vi "Heartbeat Service.vi"() -> ()   [LabVIEW 2015]
doc: "This VeriStand service checks to see if the daemon associated with the Host Hearbeat custom device is running. If the daemon is running, the service does nothing. If the deamon isn't running, the service launches the daemon. The service checks daemon status only once then ends execution."
uses:
  NationalInstruments.VeriStand.SystemStorage
  Shared/Constants.vi
  Shared/Host Heartbeat Shared.lvlib
panel:
  in  "NIVS.System Definition Root":refnum<k24>
  in  "NIVS.Gateway IP Address":string
  # "These controls are written to by name when VeriStand \nlaunches the service. DO NOT modify their names"
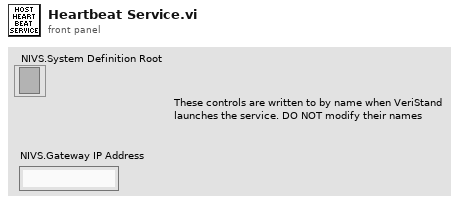
[diagram p1: front panel]
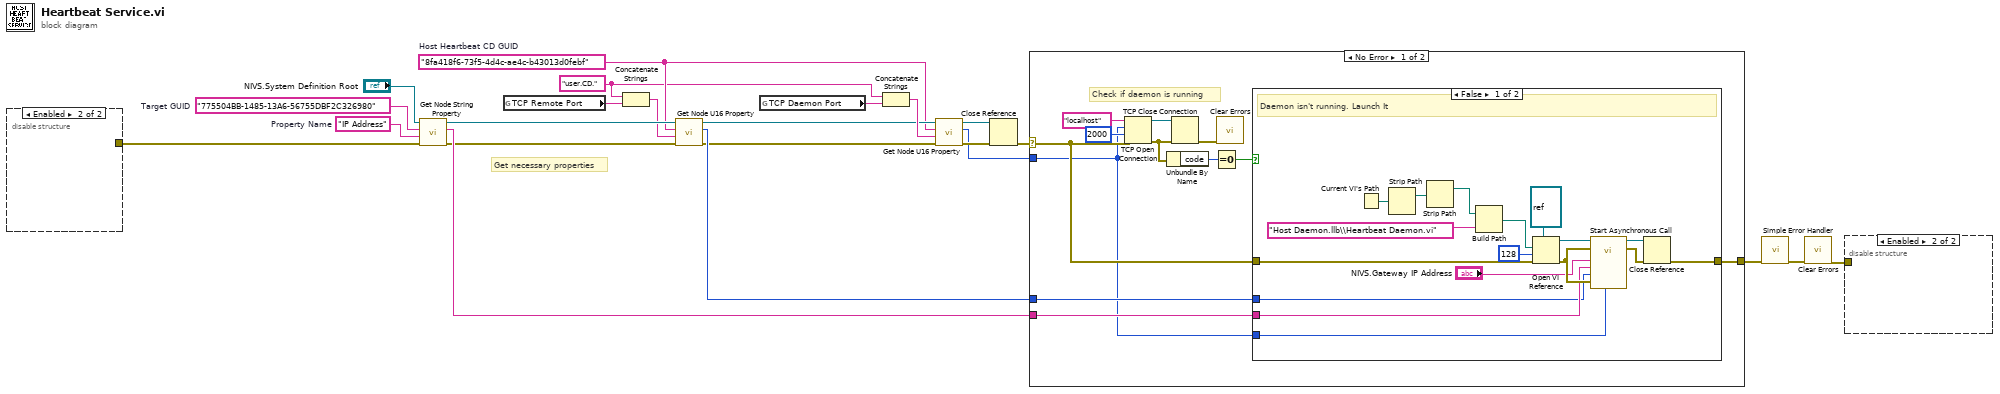
[diagram p0: block diagram]
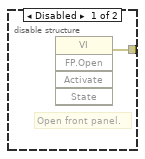
[diagram p2: hidden frame]
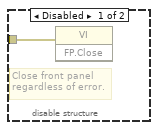
[diagram p3: hidden frame]
diagram:
  w2 = "8fa418f6-73f5-4d4c-ae4c-b43013d0febf"  # Host Heartbeat CD GUID
  w15 = "775504BB-1485-13A6-56755DBF2C326980"  # Target GUID
  w1 = "user.CD." ("string")
  w23 = "IP Address"  # Property Name
  # "Get necessary properties"
  n1 = disable-structure shown="Enabled" {
    disable-tunnel: [w24 _] -> w19
    frame Disabled {
      # "Open front panel."
      n2 = invoke class="VI" method="FP.Open"() -> (error out=w24:errorcluster)  [unwired: 5 in, 4 out]
    }
    frame Enabled {
    }
  }
  n3 = call "Get Node String Property.vi"("Error In"=w19, "Property Name"=w23, "Node GUID"=w15, "Root .NET Ref In"="NIVS.System Definition Root") -> ("Error Out"=w13:errorcluster, "Property"=w22:string, "Root .NET Ref Out"=w14:refnum<k24>)  [unwired: 5 in]
  n4 = global read "Constants.vi" "TCP Remote Port"() -> (w21:string)
  n5 = Concatenate Strings(w1, w21) -> (w10:string)
  n6 = call "Get Node U16 Property.vi"("Error In"=w13, "Property Name"=w10, "Node GUID"=w2, "Root .NET Ref In"=w14) -> ("Error Out"=w6:errorcluster, "Property"=w12:u16, "Root .NET Ref Out"=w7:refnum<k24>)  [unwired: 5 in]
  n7 = global read "Constants.vi" "TCP Daemon Port"() -> (w8:string)
  n8 = Concatenate Strings(w1, w8) -> (w9:string)
  n9 = call "Get Node U16 Property.vi"("Error In"=w6, "Property Name"=w9, "Node GUID"=w2, "Root .NET Ref In"=w7) -> ("Error Out"=w4:errorcluster, "Property"=w3:u16, "Root .NET Ref Out"=w5:refnum<k24>)  [unwired: 5 in]
  n10 = Close Reference(reference=w5, error in (no error)=w4) -> (error out=w11:errorcluster)
  n11 = case shown="No Error" w11 {
    selector: w11 -> [w27 w55]
    tunnel: [w29 w55] -> w16
    tunnel: w22 -> [w28 _]
    tunnel: w12 -> [w26 _]
    tunnel: w3 -> [w25 _]
    frame No Error {
      # "Check if daemon is running"
      n12 = TCP Open Connection(address="localhost", remote port or service name=w25, timeout ms (60000)=2000, error in (no error)=w27) -> (connection ID=w34:refnum<k5>, error out=w32:errorcluster)  [unwired: 1 in]
      n13 = Unbundle By Name(w32) -> ("code"=w31:i32)
      n14 = TCP Close Connection(connection ID=w34, error in (no error)=w32) -> (error out=w33:errorcluster)  [unwired: 1 in, 1 out]
      n15 = Equal To 0?(x=w31) -> (x = 0?=w30:bool)
      n16 = call <vilib>:"Clear Errors.vi"("error in (no error)"=w33) -> ()  [unwired: 5 in, 2 out]
      n17 = case shown="False" w30 {
        tunnel: [w41 w54] -> w29
        tunnel: w28 -> [w40 _]
        tunnel: w26 -> [w39 _]
        tunnel: w27 -> [w38 w54]
        tunnel: w25 -> [w37 _]
        frame False {
          # "Daemon isn't running. Launch It"
          n18 = Current VI's Path() -> (path=w46:path)
          n19 = Strip Path(path=w46) -> (stripped path=w45:path)  [unwired: 1 out]
          n20 = Strip Path(path=w45) -> (stripped path=w44:path)  [unwired: 1 out]
          n21 = Build Path(base path=w44, name or relative path="Host Daemon.llb\\Heartbeat Daemon.vi") -> (appended path=w47:path)
          n22 = Open VI Reference(type specifier VI Refnum (for type only)=refnum<vi> refnum, vi path=w47, options=128, error in (no error)=w38) -> (vi reference=w52:refnum<vi>, error out=w50:errorcluster)  [unwired: 2 in]
          n23 = call-by-ref "Start Asynchronous Call"(reference=w52, error in=w50, "Local Daemon Port"=w37, "Error In"=w50, "Remote Port"=w39, "Target IP"=w40, "NIVS.Gateway IP Address"="NIVS.Gateway IP Address") -> (reference out=w48:refnum<vi>, error out=w49:errorcluster)  [unwired: 7 in]
          n24 = Close Reference(reference=w48, error in (no error)=w49) -> (error out=w41:errorcluster)
        }
        frame True {
          # "Daemon is running. Do Nothing"
        }
      }
    }
    frame Error {
    }
  }
  n25 = call <vilib>:"Simple Error Handler.vi"("error in (no error)"=w16) -> ("error out"=w18:errorcluster)  [unwired: 4 in, 4 out]
  n26 = call <vilib>:"Clear Errors.vi"("error in (no error)"=w18) -> ("error out"=w17:errorcluster)  [unwired: 5 in, 1 out]
  n27 = disable-structure shown="Enabled" {
    disable-tunnel: w17 -> [w56 _]
    frame Disabled {
      # "Close front panel\nregardless of error."
      n28 = invoke class="VI" method="FP.Close"(error in=w56) -> ()  [unwired: 2 in, 3 out]
    }
    frame Enabled {
    }
  }
